vi "_RT_CtrlLoop_D999_ValueConvNormStr.vi"(7 "AI_Param":T1(array[cluster])=[{"Label"="", "MultiValue"=1.0, "AddValue"=0.0}, {"Label"="", "MultiValue"=1.0, "AddValue"=0.0}, {"Label"="", "MultiValue"=1.0, "AddValue"=0.0}, {"Label"="", "MultiValue"=1.0, "AddValue"=0.0}, {"Label"="", "MultiValue"=1.0, "AddValue"=0.0}, {"Label"="", "MultiValue"=1.0, "AddValue"=0.0}, {"Label"="", "MultiValue"=1.0, "AddValue"=0.0}, {"Label"="", "MultiValue"=1.0, "AddValue"=0.0}, {"Label"="", "MultiValue"=1.0, "AddValue"=0.0}, {"Label"="", "MultiValue"=1.0, "AddValue"=0.0}, {"Label"="", "MultiValue"=1.0, "AddValue"=0.0}, {"Label"="", "MultiValue"=1.0, "AddValue"=0.0}], 8 "error in (no error)":errorcluster, 10 "appended array":i32[](array[numeric])) -> (0 "error out":errorcluster, 2 "EC Format":T2)   [LabVIEW 2018]
uses:
  PublicSubVI/Ctl/_ctl_RT_D999_Format.ctl
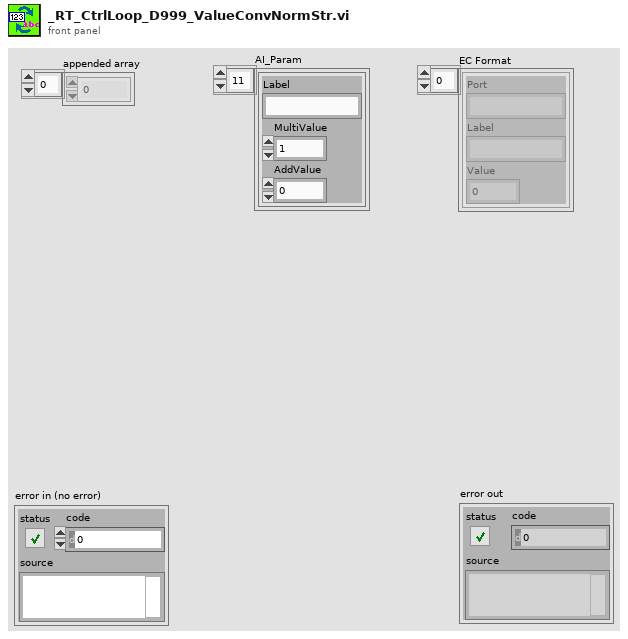
[diagram p1: front panel]
types:
  T1 = cluster{"Label":string, "MultiValue":dbl, "AddValue":dbl}[]
  T2 = typedef "_ctl_RT_D999_Format.ctl" = cluster{"Port":string, "Label":string, "Value":dbl}[]
  T3 = cluster{"Port":string, "Label":string, "Value":dbl}
  T4 = cluster{"Port":string, "Label":string, "Value":dbl}[]
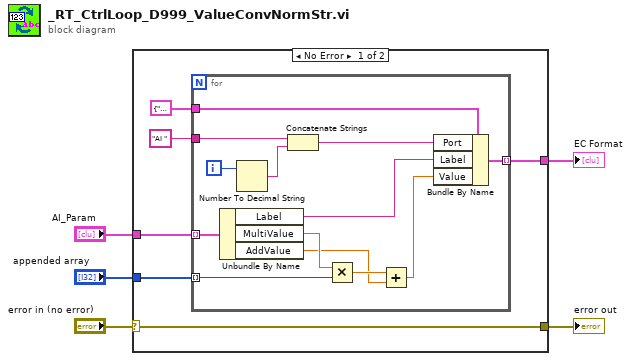
[diagram p0: block diagram]
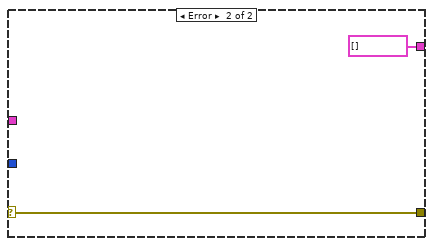
[diagram p2: hidden frame]
diagram:
  n1 = case shown="No Error" "error in (no error)" {
    selector: "error in (no error)" -> [w8 w26]
    tunnel: [w9 T4 []] -> w5
    tunnel: [w8 w26] -> w3
    tunnel: "AI_Param" -> [w7 _]
    tunnel: "appended array" -> [w6 _]
    frame No Error {
      n2 = for {
        tunnel: w7 -> [w23] mode=indexing
        tunnel: w6 -> [w20] mode=indexing
        tunnel: T3 {"Port"="", "Label"="", "Value"=0.0} -> [w16]
        tunnel: "AI " -> [w18]
        tunnel: [w12] -> w9 mode=indexing
        i -> [w19]
        n3 = Unbundle By Name(w23) -> ("Label"=w14:string, "MultiValue"=w22:dbl, "AddValue"=w21:dbl)
        n4 = Number To Decimal String(number=w19) -> (decimal integer string=w17:string)  [unwired: 1 in]
        n5 = Concatenate Strings(w18, w17) -> (w15:string)
        n6 = Multiply(x=w22, y=w20) -> (x*y=w24:dbl)
        n7 = Add(x=w24, y=w21) -> (x+y=w13:dbl)
        n8 = Bundle By Name(cluster=w16, "Port"=w15, "Label"=w14, "Value"=w13) -> (w12:T3)
      }
    }
    frame Error {
    }
  }
  "error out" <- w3
  "EC Format" <- w5
